vi "5785_2_x_200MHz_multi emitter.vi"() -> ()   [LabVIEW 2021]
uses:
  <instrlib>/_niInstr/Streaming/v1/Common/Stream State.ctl
  <vilib>/Platform/TimedLoop/XDataNode/timing_clust.ctl
  <vilib>/Platform/TimedLoop/XDataNode/nitl_modes.ctl
  <vilib>/Platform/TimedLoop/XDataNode/wakeup.ctl
  <instrlib>/FlexRIO/API/FPGA/v1/Types/Start Trigger IO Resources.ctl
  <vilib>/rvi/Emulation/niFpgaSctlEmulationGetInTimedLoop.vi
  <vilib>/rvi/Emulation/niFpgaEmulationReportErrorSimple.vi
  <vilib>/rvi/Emulation/niFpgaGetClockAttributes.vi
  <vilib>/rvi/Emulation/niFpgaCriticalErrorInLSC.vi
  7192f61d-e408-4cca-baff-cb10c33219c0.vi
  <vilib>/rvi/interface/RandomDataEmulation/nirviRandomDataMultiElementFPGAFIFO.vi
  <instcachedir>/0/nirviRandomDataMultiElementFPGAFIFO_3E9965BA1FAD4E7B8DABA31768A09B1F.lvgen/nirviRandomDataMultiElementFPGAFIFO_3E9965BA1FAD4E7B8DABA31768A09B1F_000.vi
  <vilib>/rvi/interface/RandomDataEmulation/niFpgaRandomDataHandleErrors.vi
  <instrlib>/_niInstr/DSP/v1/FPGA/Public/Sub VIs/HB Interpolator/Halfband Interpolator - IQ - 1 SPC - 2x OC.vi
  <instrlib>/_niInstr/DSP/v1/FPGA/Public/Sub VIs/HB Interpolator/Halfband Interpolator - IQ - 2 SPC - 2x OC.vi
  <instrlib>/_niInstr/DSP/v1/FPGA/Public/Sub VIs/HB Interpolator/Halfband Interpolator - IQ - 4 SPC - 2x OC.vi
  <instrlib>/_niInstr/DSP/v1/FPGA/Public/Sub VIs/HB Interpolator/Halfband Interpolator - IQ - 8 SPC - 2x OC.vi
  <instrlib>/_niInstr/DSP/v1/FPGA/Public/Sub VIs/Frequency Shift/Frequency Shift - 16 spc.vi
  <vilib>/rvi/eio/common/nirviEmuTemplateMethod_errors.vi
  <vilib>/Platform/TimedLoop/XDataNode/XDataNode.xnode
  <vilib>/rvi/DataTransferAndStorage/Container/XNode/niFpgaContainer.xnode
  <vilib>/rvi/interface/RandomDataEmulation/nirviRandomDataFpgaMultiElementTemplate.vi
  <vilib>/eio/EIONode/EIONode.xnode
  <vilib>/Platform/TimedLoop/XDataNode/XDNodeRunTimeDep.lvlib
  <instrlib>/_niInstr/Streaming/v1/FPGA/niInstr Streaming v1 FPGA.lvlib
  <instrlib>/FlexRIO/API/FPGA/v1/FlexRIO API FPGA v1.lvlib
  <instrlib>/FlexRIO/API/FPGA/v1/IO/NI5785/FlexRIO 5785 FPGA v1.lvlib
  <instrlib>/_niInstr/DSP/v1/FPGA/niInstr DSP v1 FPGA.lvlib
  <instrlib>/_niInstr/Basic Elements/v1/FPGA/niInstr Basic Elements v1 FPGA.lvlib
  <instrlib>/_niInstr/Streaming/v1/Common/niInstr Streaming v1 Common.lvlib
panel:
  out "clock fail":bool
  out "dds free 2":bool[](array[boolean])
  out "dds free":bool[](array[boolean])
  out "pulse transmitted 2":u32
  out "pulse transmitted":u32
  out "fpga clock 2":u64
  out "fpga clock":u64
  in  "reset system clock":bool
  in  "frequency shift 1":fxp<+/-,48,0>
  in  "User-defined Start Trigger - AO":bool
  in  "flexrio.trigger.start.cfg 1":u16
  out "written elements":u64
  out "IO Socket\\AO Ready For Input":bool
  in  "stream.request state 1":T1
  in  "stream.num samples 1":u64
  out "stream.metadata 1":u64
  out "stream.samples transferred 1":u64
  out "stream.state 1":T1
  out "flexrio.module.io ready 0":bool
  out "flexrio.module.io error 0":i32
  out "flexrio.module.data valid 0":bool
  # "Data Path Configuration"
  # "AI Trigger Configuration"
  # "AI Stream Configuration"
  # "AO Stream Configuration"
  # "Module Status"
  # "AO Buffer Configuration"
  # "Device Utilization\n---------------------------\nTotal Slices: 62.6% (18977 out of 30300)\nSlice Registers: 23.8% (115206 out of 484800)\nSlice LUTs: 38.2% (92532 out of 242400)\nBlock RAMs: 56.8% (341 out of 600)\nDSP48s: 0.3% (6 out of 1920)\n\nNote: Utilization numbers are for the KU040. Exact values will vary for the KU060 and KU035."
  # "User-defined Controls"
  # "AO Trigger Configuration"
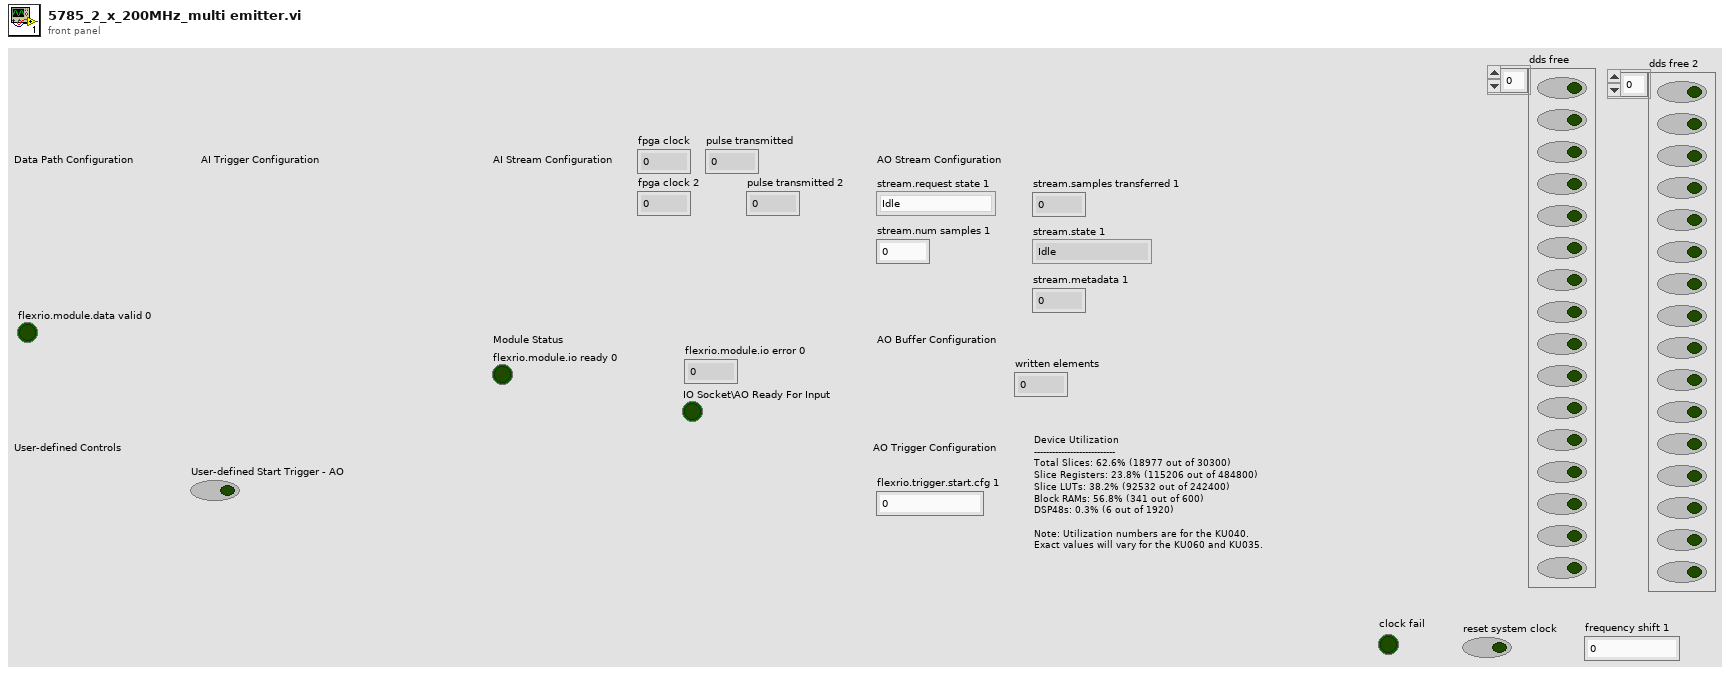
[diagram p1: front panel]
types:
  T1 = typedef "niInstr Streaming v1 Common.lvlib/Stream State.ctl" = enum8{"Idle", "Finite Transfer", "Continuous", "Done", "Error", "Not Ready", "Cancel"}
  T2 = typedef "XDNodeRunTimeDep.lvlib/timing_clust.ctl" = cluster{"Expected End [f-1]":u64, "Actual End [f-1]":u64, "Finished Late? [f-1]":bool, "Expected End [i-1]":u64, "Actual End [i-1]":u64, "Finished Late? [i-1]":bool, "Expected Start [i]":u64, "Actual Start [i]":u64, "Expected Start [f]":u64, "Actual Start [f]":u64, "Source Name":string, "Structure Name":string, "Period":i64, "Deadline":i64, "Offset":i64, "Start":i64, "Priority":i32, "Timeout":i32, "Mode":T3, "Wakeup Reason":T4, "Error":errorcluster, "Source Type":string, "Secondary Source Type":string, "Global End Time":u64, "Global Start Time":u64, "Frame Duration":u64, "Iteration Duration":u64, "Assigned CPU":i32, "I/O Scan Engine Mode":u32}
  T3 = typedef "XDNodeRunTimeDep.lvlib/nitl_modes.ctl" = enum32{"No Change", "Process missed periods, maintain original phase", "Discard missed periods, maintain original phase", "Process missed periods, ignore original phase", "Discard missed periods, ignore original phase"}
  T4 = typedef "XDNodeRunTimeDep.lvlib/wakeup.ctl" = enum32{"Normal", "Aborted", "Asynchronous wakeup", "Timing source error", "Timed loop error", "Timeout"}
  T5 = typedef "FlexRIO API FPGA v1.lvlib/Start Trigger IO Resources.ctl" = cluster{"start trigger":refnum<k21>, "started event":refnum<k21>, "start trigger for export":refnum<k21>, "start trigger for tclk":refnum<k21>}
  T6 = typedef "FlexRIO API FPGA v1.lvlib/Start Trigger Control.ctl" = cluster{"arm start":bool, "done":bool}
  T7 = typedef "niInstr DSP v1 Shared.lvlib/IQ Data.ctl" = cluster{"I":fxp<+/-,18,1>, "Q":fxp<+/-,18,1>, "overflow":bool}
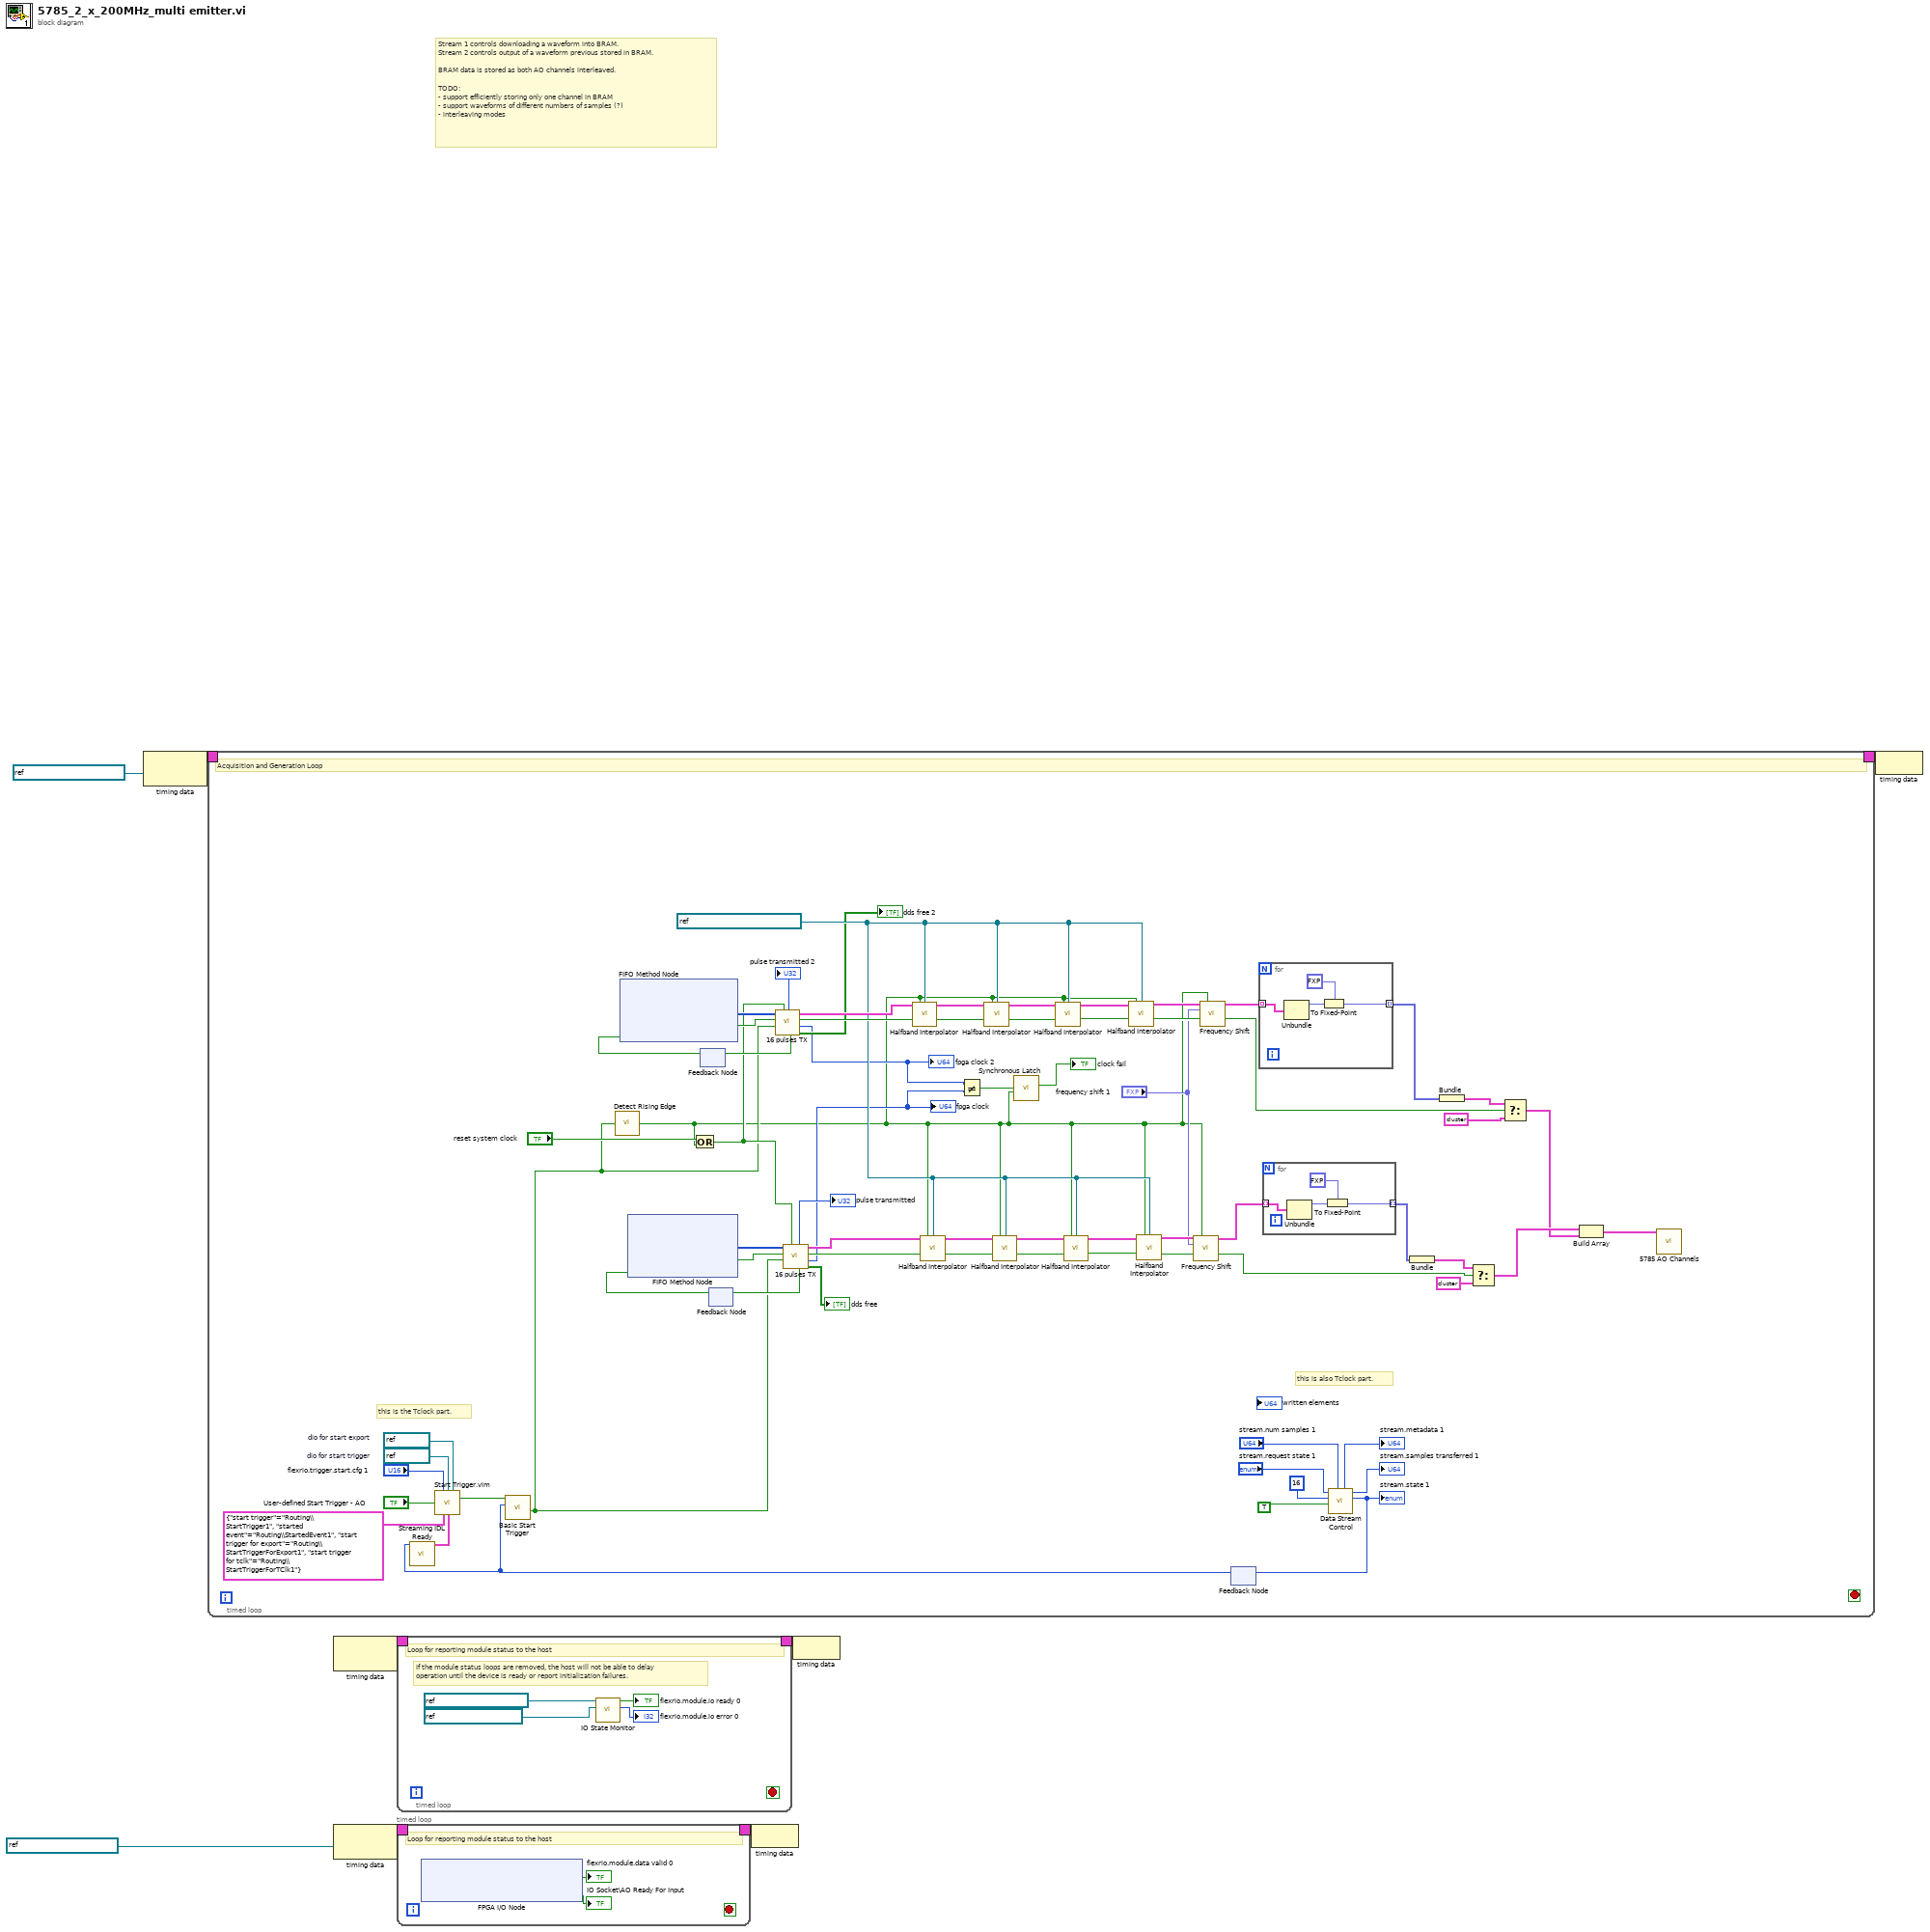
[diagram p0: block diagram]
diagram:
  # "Stream 1 controls downloading a waveform into BRAM.\nStream 2 controls output of a waveform previous stored in BRAM.\n\nBRAM data is stored as both AO channels interleaved.\n\nTODO:\n- support efficiently storing only one channel in BRAM\n- support waveforms of different numbers of samples (?)\n- interleaving modes"
  n1 = node-c288(refnum<k21> "IO Socket\\Data Clock" ("Source Name")) -> (w8:T2)
  n2 = timed-loop {
    timing: w8 -> [_]
    timing-out: [_] -> w7
    stop <- _ stop-if-true
    w35 = refnum<k21> "IO Socket\\Data Clock 2x" ("Source Name")
    w67 = refnum<k21> "DIO 2"  # dio for start trigger
    w66 = refnum<k21> "DIO 3"  # dio for start export
    # "this is also Tclock part."
    # "this is the Tclock part."
    # "Acquisition and Generation Loop"
    n3 = feedback #1() -> (w47:bool)  [unwired: 1 in]
    n4 = xnode ("FIFO Method Node")("Ready for Output"=w47) -> ("Element"=w50:u64[], "Output Valid"=w45:bool)  [unwired: 1 in, 1 out]
    n5 = feedback #2() -> (w52:bool)  [unwired: 1 in]
    n6 = xnode ("FIFO Method Node")("Ready for Output"=w52) -> ("Element"=w51:u64[], "Output Valid"=w29:bool)  [unwired: 1 in, 1 out]
    n7 = feedback #3() -> (w64:T1)  [unwired: 1 in]
    n8 = call <instrlib>:"Streaming IDL Ready.vi"("stream.state"=w64) -> ("start trigger control"=w69:T6)  [unwired: 10 in]
    n9 = call "Start Trigger.vim"("flexrio.trigger.start.cfg 0"="flexrio.trigger.start.cfg 1", "dio start"=w67, "dio for start export"=w66, "user-defined start trigger"="User-defined Start Trigger - AO", "trigger io resources"=T5 {"start trigger"="Routing\\StartTrigger1", "started event"="Routing\\StartedEvent1", "start trigger for export"="Routing\\StartTriggerForExport1", "start trigger for tclk"="Routing\\StartTriggerForTClk1"}, "start trigger control"=w69) -> ("conditioned start trigger"=w68:bool)  [unwired: 7 in, 2 out]
    n10 = call <instrlib>:"Basic Start Trigger.vi"("stream.state"=w64, "start trigger"=w68) -> ("data valid"=w32:bool)  [unwired: 9 in]
    n11 = call <instrlib>:"Detect Rising Edge.vi"("signal"=w32) -> ("edge detected"=w10:bool)  [unwired: 14 in]
    n12 = Or(x="reset system clock", y=w10) -> (x .or. y?=w33:bool)
    n13 = call "16 pulses TX.vi"("reset system clock"=w33, "IQ_run"=w32, "PDW input Valid"=w45, "array PDW"=w50) -> ("dds free"=→"dds free 2":bool[], "fpga clock"=w13:u64, "output valid"=w49:bool, "RF OUT"=w48:T7, "ready for input"=w46:bool, "pulse transmitted"=→"pulse transmitted 2":u32)  [unwired: 2 in]
    "fpga clock 2" <- w13
    n14 = feedback-in #1(w46) -> ()
    n15 = call "16 pulses TX.vi"("reset system clock"=w33, "IQ_run"=w32, "PDW input Valid"=w29, "array PDW"=w51) -> ("dds free"=→"dds free":bool[], "fpga clock"=w12:u64, "output valid"=w24:bool, "RF OUT"=w25:T7, "ready for input"=w53:bool, "pulse transmitted"=→"pulse transmitted":u32)  [unwired: 2 in]
    "fpga clock" <- w12
    n16 = feedback-in #2(w53) -> ()
    n17 = call-poly <instrlib>:"Halfband Interpolator.vi"("data in"=w48, "reset"=w10, "clock x 2"=w35, "input valid"=w49) -> ("data out"=w36:T7[], "output valid"=w44:bool)  [unwired: 8 in, 2 out]
    n18 = call-poly <instrlib>:"Halfband Interpolator.vi"("data in"=w25, "reset"=w10, "clock x 2"=w35, "input valid"=w24) -> ("data out"=w62:T7[], "output valid"=w54:bool)  [unwired: 8 in, 2 out]
    n19 = Not Equal?(x=w13, y=w12) -> (x != y?=w11:bool)
    n20 = call-poly <instrlib>:"Halfband Interpolator.vi"("data in"=w36, "reset"=w10, "clock x 2"=w35, "input valid"=w44) -> ("data out"=w37:T7[], "output valid"=w43:bool)  [unwired: 8 in, 2 out]
    n21 = call-poly <instrlib>:"Halfband Interpolator.vi"("data in"=w62, "reset"=w10, "clock x 2"=w35, "input valid"=w54) -> ("data out"=w61:T7[], "output valid"=w55:bool)  [unwired: 8 in, 2 out]
    n22 = call <instrlib>:"Synchronous Latch.vi"("clear"=w10, "set"=w11) -> ("out"=→"clock fail":bool)  [unwired: 9 in]
    n23 = call-poly <instrlib>:"Halfband Interpolator.vi"("data in"=w37, "reset"=w10, "clock x 2"=w35, "input valid"=w43) -> ("data out"=w38:T7[], "output valid"=w42:bool)  [unwired: 8 in, 2 out]
    n24 = call-poly <instrlib>:"Halfband Interpolator.vi"("data in"=w61, "reset"=w10, "clock x 2"=w35, "input valid"=w55) -> ("data out"=w60:T7[], "output valid"=w56:bool)  [unwired: 8 in, 2 out]
    n25 = call-poly <instrlib>:"Halfband Interpolator.vi"("data in"=w38, "reset"=w10, "clock x 2"=w35, "input valid"=w42) -> ("data out"=w39:T7[], "output valid"=w41:bool)  [unwired: 8 in, 2 out]
    n26 = call-poly <instrlib>:"Halfband Interpolator.vi"("data in"=w60, "reset"=w10, "clock x 2"=w35, "input valid"=w56) -> ("data out"=w59:T7[], "output valid"=w57:bool)  [unwired: 8 in, 2 out]
    n27 = call-poly <instrlib>:"Frequency Shift.vi"("data in"=w59, "reset"=w10, "frequency shift"="frequency shift 1", "input valid"=w57) -> ("data out"=w58:T7[], "output valid"=w22:bool)  [unwired: 8 in, 2 out]
    n28 = call-poly <instrlib>:"Frequency Shift.vi"("data in"=w39, "reset"=w10, "frequency shift"="frequency shift 1", "input valid"=w41) -> ("data out"=w40:T7[], "output valid"=w15:bool)  [unwired: 8 in, 2 out]
    n29 = for {
      tunnel: w40 -> [w82] mode=indexing
      tunnel: [w79] -> w27 mode=indexing
      n30 = Unbundle(w82) -> ("I"=w81:fxp<+/-,18,1>)  [unwired: 2 out]
      n31 = To Fixed-Point(fixed-point type=fxp<+/-,12,1> 0.0 ("element"), number=w81) -> (fixed-point=w79:fxp<+/-,12,1>)
    }
    n32 = for {
      tunnel: w58 -> [w86] mode=indexing
      tunnel: [w83] -> w28 mode=indexing
      n33 = Unbundle(w86) -> ("I"=w85:fxp<+/-,18,1>)  [unwired: 2 out]
      n34 = To Fixed-Point(fixed-point type=fxp<+/-,12,1> 0.0 ("element"), number=w85) -> (fixed-point=w83:fxp<+/-,12,1>)
    }
    n35 = call <instrlib>:"Data Stream Control.vi"("stream.num samples 0"="stream.num samples 1", "data valid"=TRUE, "element count"=u16 16, "stream.request state 0"="stream.request state 1") -> ("stream.state 0"=w71:T1, "stream.samples transferred 0"=→"stream.samples transferred 1":u64, "stream.metadata 0"=→"stream.metadata 1":u64)  [unwired: 3 in, 2 out]
    "stream.state 1" <- w71
    n36 = feedback-in #3(w71) -> ()
    n37 = Bundle(w28) -> (w21:cluster{fxp<+/-,12,1>[]})  [unwired: 1 in]
    n38 = Bundle(w27) -> (w17:cluster{fxp<+/-,12,1>[]})  [unwired: 1 in]
    n39 = Select(t=w21, s=w22, f=cluster{fxp<+/-,12,1>[]} {[0.0, 0.0, 0.0, 0.0, 0.0, 0.0, 0.0, 0.0, 0.0, 0.0, 0.0, 0.0, 0.0, 0.0, 0.0, 0.0]}) -> (s? t:f=w20:cluster{fxp<+/-,12,1>[]})
    n40 = Select(t=w17, s=w15, f=cluster{fxp<+/-,12,1>[]} {[0.0, 0.0, 0.0, 0.0, 0.0, 0.0, 0.0, 0.0, 0.0, 0.0, 0.0, 0.0, 0.0, 0.0, 0.0, 0.0]}) -> (s? t:f=w16:cluster{fxp<+/-,12,1>[]})
    n41 = Build Array(w20, w16) -> (w76:cluster{fxp<+/-,12,1>[]}[])
    n42 = call <instrlib>:"5785 AO Channels.vi"("all channels"=w76) -> ()  [unwired: 15 in]
  }
  n43 = node-c288() -> (w5:T2)  [unwired: 1 in]
  n44 = node-c288(refnum<k21> "IO Socket\\Data Clock" ("Source Name")) -> (w3:T2)
  n45 = timed-loop {
    timing: w5 -> [_]
    timing-out: [_] -> w4
    stop <- _ stop-if-true
    # "If the module status loops are removed, the host will not be able to delay operation until the device is ready or report initialization failures."
    # "Loop for reporting module status to the host"
    n46 = call <instrlib>:"IO State Monitor.vi"("io error resource"=refnum<k21> "IO Socket\\IO Error" ("FPGA I/O In"), "io ready resource"=refnum<k21> "IO Socket\\IO Ready" ("FPGA I/O In")) -> ("flexrio.module.io error 0"=→"flexrio.module.io error 0":i32, "flexrio.module.io ready 0"=→"flexrio.module.io ready 0":bool)  [unwired: 8 in]
  }
  n47 = timed-loop {
    timing: w3 -> [_]
    timing-out: [_] -> w2
    stop <- _ stop-if-true
    # "Loop for reporting module status to the host"
    n48 = xnode "FPGA I/O Node"() -> ("IO Socket\\AI Data Valid"=→"flexrio.module.data valid 0":bool, "IO Socket\\AO Ready For Input"=→"IO Socket\\AO Ready For Input":bool)  [unwired: 2 in, 2 out]
  }
  n49 = node-c288(w2) -> ()
  n50 = node-c288(w4) -> ()
  n51 = node-c288(w7) -> ()
